vi "ColumnHeadersSet.vi"() -> (0 "error out":errorcluster)   [LabVIEW 2019, in "ResultTreeTest.lvlib" / "CreateResultTree.lvlib"]
uses:
  a00fc3d9-dfa3-46aa-b3da-e1bcdc76d972.vi
  Constraint/IsEqual/Create.vi
  Constraint/IsEqual/IsEqual.lvclass
  CreateResultTree.lvlib
  ResultTree/ResultTree.lvclass
panel:
  in  "Tree":string(tree)
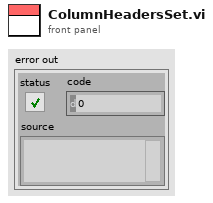
[diagram p1: front panel]
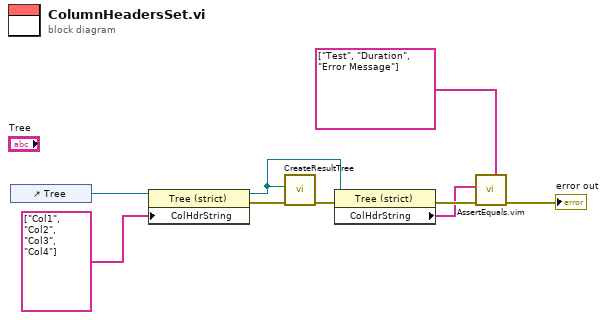
[diagram p0: block diagram]
diagram:
  n1 = control-ref of="Tree"() -> (w9:refnum<vi>)
  n2 = property class="Tree (strict)"(reference=w9, "ColHdrString"=string[] ["Col1", "Col2", "Col3", "Col4"] ("Column Header Strings[]")) -> (reference out=w6:refnum<vi>, error out=w8:errorcluster)  [unwired: 1 in]
  n3 = call "CreateResultTree.vi"("error in (no error)"=w8, "Tree Refnum"=w6) -> ("error out"=w7:errorcluster)  [unwired: 8 in, 1 out]
  n4 = property class="Tree (strict)"(reference=w6, error in=w7) -> (error out=w5:errorcluster, "ColHdrString"=w2:string[])  [unwired: 1 out]
  n5 = call "AssertEquals.vim"("Expected"=string[] ["Test", "Duration", "Error Message"] ("Column Header Strings[]"), "error in (no error)"=w5, "Actual"=w2) -> ("error out"=→"error out":errorcluster)  [unwired: 8 in]
